vi "RH_DCPower_Configure.vi"(6 "output terminal":tag, 7 "DCPower_Parameters":T1={"Output"=enum."DC Voltage", "Current_range"=0.0, "Current"=0.0, "Voltage_range"=0.0, "Voltage"=0.0, "Aperture_time"=0.0, "Source Delay"=0.0, "Sense"=1008} {"Source Delay" format="%.6p"; "Sense" items=["Local"=1008, "Remote"=1009]; "Aperture_time" format="%.6p"; "Current_range" format="%.6p"; "Current" format="%.6p"; "Voltage_range" format="%.6p"; "Voltage" format="%.6p"}, 8 "error in (no error)":errorcluster, 9 "trigger out?":bool, 10 "channel name":string, 11 "DCPower Session In":refnum<k15>) -> (0 "error out":errorcluster, 3 "DCPower Session Out":refnum<k15>)   [LabVIEW 2023, in "ResourceHandling.lvlib"]
doc: "Config SMU/PS channel in DC Voltage or DC Current mode, exporting Start Trigger and setting the Aperture Time"
uses:
  ResourceHandling.lvlib
  TypeDefs/RH_DCPower_Parameters.ctl
  <instrlib>/niDCPower/nidcpower.llb/niDCPower Source Mode.ctl
  <instrlib>/niDCPower/nidcpower.llb/niDCPower Output Function.ctl
  <instrlib>/niDCPower/nidcpower.llb/niDCPower Export Signal - Signal.ctl
  <instrlib>/niDCPower/nidcpower.llb/niDCPower Aperture Time Units.ctl
  <instrlib>/niDCPower/nidcpower.llb/niDCPower Disable Start Trigger With Channels.vi
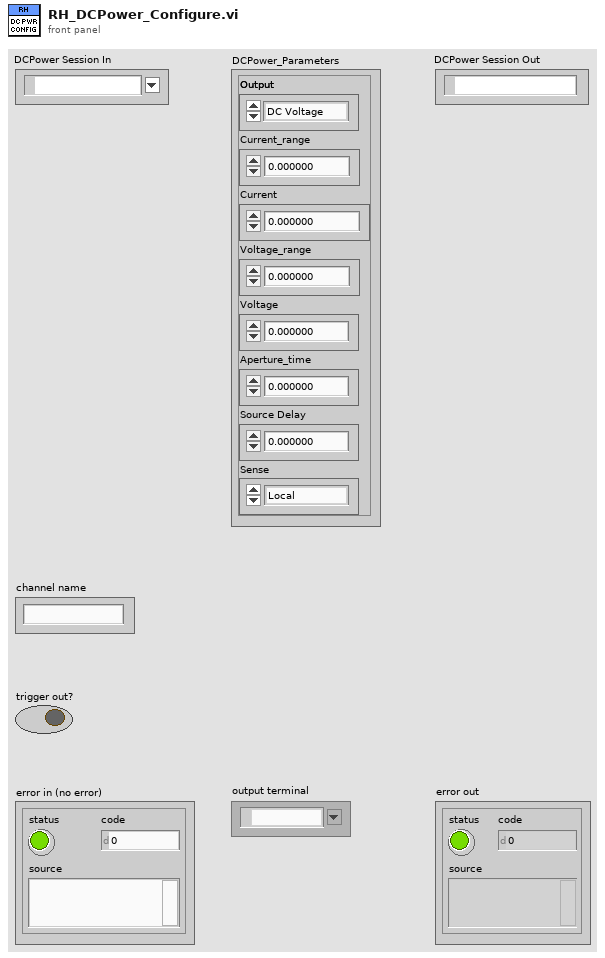
[diagram p1: front panel]
types:
  T1 = typedef "ResourceHandling.lvlib/RH_DCPower_Parameters.ctl" = cluster{"Output":enum16{"DC Voltage", "DC Current"}, "Current_range":dbl, "Current":dbl, "Voltage_range":dbl, "Voltage":dbl, "Aperture_time":dbl, "Source Delay":dbl, "Sense":i32}
  T2 = typedef "niDCPower Source Mode.ctl" = i32
  T3 = typedef "niDCPower Output Function.ctl" = i32
  T4 = typedef "niDCPower Export Signal - Signal.ctl" = i32
  T5 = typedef "niDCPower Aperture Time Units.ctl" = i32
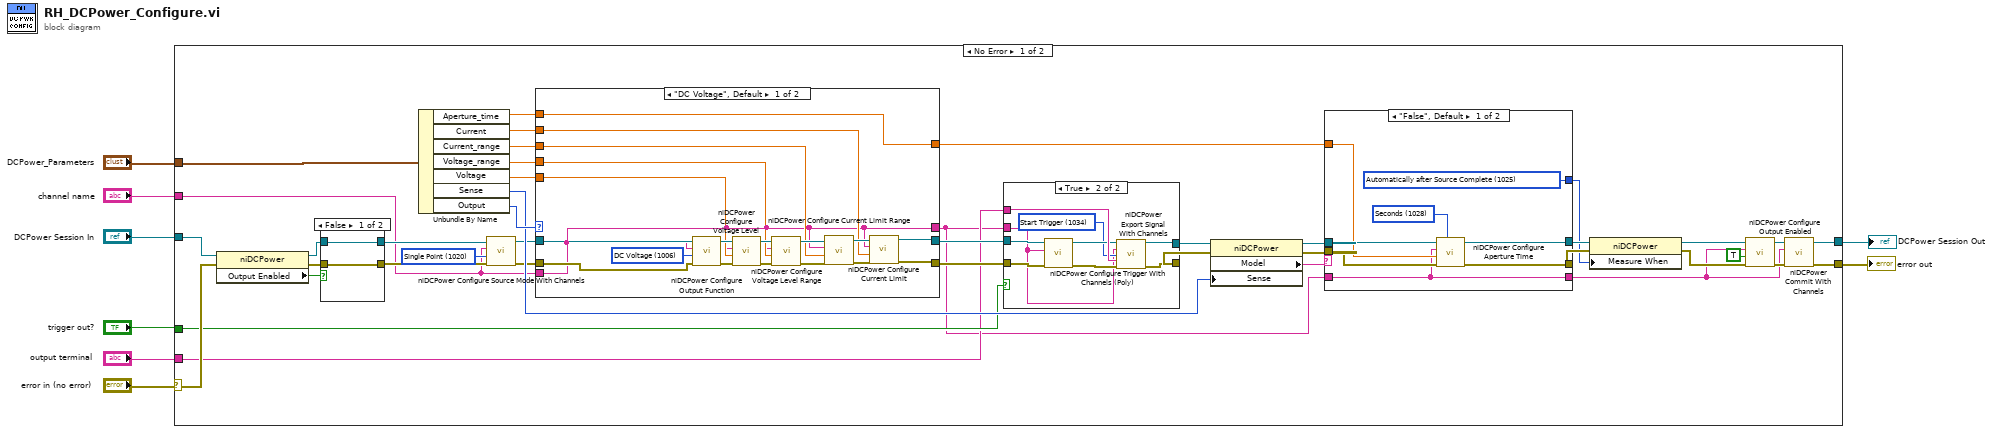
[diagram p0: block diagram]
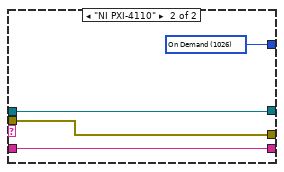
[diagram p2: hidden frame]
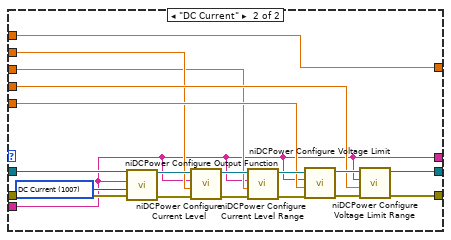
[diagram p4: hidden frame]
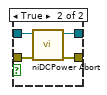
[diagram p5: hidden frame]
diagram:
  n1 = case shown="No Error" "error in (no error)" {
    selector: "error in (no error)" -> [w31 w118]
    tunnel: "DCPower_Parameters" -> [w35 _]
    tunnel: "DCPower Session In" -> [w34 w117]
    tunnel: [w33 w117] -> w1
    tunnel: [w32 w118] -> w7
    tunnel: "channel name" -> [w10 _]
    tunnel: "trigger out?" -> [w19 _]
    tunnel: "output terminal" -> [w18 _]
    frame No Error {
      w24 = T2 1020 items=["Single Point"=1020, "Sequence"=1021] ("source mode")
      n2 = property class="niDCPower"(reference=w34, error in=w31) -> (reference out=w48:refnum<k15>, error out=w49:errorcluster, "Output Enabled"=w47:bool)
      n3 = case shown="False" w47 {
        tunnel: w48 -> [w112 w116]
        tunnel: w49 -> [w111 w115]
        tunnel: [w112 w114] -> w28
        tunnel: [w111 w113] -> w26
        frame False {
        }
        frame True {
          n4 = call <instrlib>:"niDCPower Abort.vi"("error in (no error)"=w115, "instrument handle"=w116) -> ("error out"=w113:errorcluster, "instrument handle out"=w114:refnum<k15>)  [unwired: 8 in]
        }
      }
      n5 = Unbundle By Name(w35) -> ("Aperture_time"=w40:dbl, "Current"=w41:dbl, "Current_range"=w42:dbl, "Voltage_range"=w43:dbl, "Voltage"=w44:dbl, "Sense"=w29:i32, "Output"=w30:enum16{"DC Voltage", "DC Current"})
      n6 = call <instrlib>:"niDCPower Configure Source Mode With Channels.vi"("error in (no error)"=w26, "source mode"=w24, "channel name"=w10, "instrument handle"=w28) -> ("error out"=w25:errorcluster, "instrument handle out"=w27:refnum<k15>)  [unwired: 6 in]
      n7 = case shown="\"DC Voltage\", Default" w30 {
        tunnel: w25 -> [w82 w102]
        tunnel: w27 -> [w83 w101]
        tunnel: [w76 w97] -> w23
        tunnel: [w75 w96] -> w21
        tunnel: w44 -> [w86 w98]
        tunnel: w43 -> [w85 w99]
        tunnel: w42 -> [w79 w93]
        tunnel: w41 -> [w74 w94]
        tunnel: w40 -> [w84 w95]
        tunnel: [w84 w95] -> w36
        tunnel: w10 -> [w73 w92]
        tunnel: [w73 w92] -> w12
        frame "DC Voltage", Default {
          w87 = T3 1006 items=["DC Voltage"=1006, "DC Current"=1007, "Pulse Voltage"=1049, "Pulse Current"=1050] ("output function")
          n8 = call <instrlib>:"niDCPower Configure Output Function.vi"("error in (no error)"=w82, "output function"=w87, "channel name"=w73, "instrument handle"=w83) -> ("error out"=w89:errorcluster, "instrument handle out"=w88:refnum<k15>)  [unwired: 6 in]
          n9 = call <instrlib>:"niDCPower Configure Voltage Level.vi"("error in (no error)"=w89, "voltage level"=w86, "channel name"=w73, "instrument handle"=w88) -> ("error out"=w91:errorcluster, "instrument handle out"=w90:refnum<k15>)  [unwired: 6 in]
          n10 = call <instrlib>:"niDCPower Configure Voltage Level Range.vi"("error in (no error)"=w91, "voltage level range"=w85, "channel name"=w73, "instrument handle"=w90) -> ("error out"=w81:errorcluster, "instrument handle out"=w80:refnum<k15>)  [unwired: 6 in]
          n11 = call <instrlib>:"niDCPower Configure Current Limit Range.vi"("error in (no error)"=w81, "current limit range"=w79, "channel name"=w73, "instrument handle"=w80) -> ("error out"=w78:errorcluster, "instrument handle out"=w77:refnum<k15>)  [unwired: 6 in]
          n12 = call <instrlib>:"niDCPower Configure Current Limit.vi"("error in (no error)"=w78, "current limit"=w74, "channel name"=w73, "instrument handle"=w77) -> ("error out"=w75:errorcluster, "instrument handle out"=w76:refnum<k15>)  [unwired: 6 in]
        }
        frame "DC Current" {
          w100 = T3 1007 items=["DC Voltage"=1006, "DC Current"=1007, "Pulse Voltage"=1049, "Pulse Current"=1050] ("output function")
          n13 = call <instrlib>:"niDCPower Configure Output Function.vi"("error in (no error)"=w102, "output function"=w100, "channel name"=w92, "instrument handle"=w101) -> ("error out"=w103:errorcluster, "instrument handle out"=w104:refnum<k15>)  [unwired: 6 in]
          n14 = call <instrlib>:"niDCPower Configure Current Level.vi"("error in (no error)"=w103, "current level"=w94, "channel name"=w92, "instrument handle"=w104) -> ("error out"=w110:errorcluster, "instrument handle out"=w109:refnum<k15>)  [unwired: 6 in]
          n15 = call <instrlib>:"niDCPower Configure Current Level Range.vi"("error in (no error)"=w110, "current level range"=w93, "channel name"=w92, "instrument handle"=w109) -> ("error out"=w108:errorcluster, "instrument handle out"=w107:refnum<k15>)  [unwired: 6 in]
          n16 = call <instrlib>:"niDCPower Configure Voltage Limit.vi"("error in (no error)"=w108, "voltage limit"=w98, "channel name"=w92, "instrument handle"=w107) -> ("error out"=w106:errorcluster, "instrument handle out"=w105:refnum<k15>)  [unwired: 6 in]
          n17 = call <instrlib>:"niDCPower Configure Voltage Limit Range.vi"("error in (no error)"=w106, "voltage limit range"=w99, "channel name"=w92, "instrument handle"=w105) -> ("error out"=w96:errorcluster, "instrument handle out"=w97:refnum<k15>)  [unwired: 6 in]
        }
      }
      n18 = case shown="True" w19 {
        tunnel: w23 -> [w63 w69]
        tunnel: [w63 w72] -> w22
        tunnel: w21 -> [w62 w67]
        tunnel: [w62 w71] -> w20
        tunnel: w18 -> [_ w70]
        tunnel: w12 -> [_ w64]
        frame False {
        }
        frame True {
          w65 = T4 1034 items=["Source Complete Event"=1030, "Measure Complete Event"=1031, "Sequence Iteration Complete Event"=1032, "Sequence Engine Done Event"=1033, "Pulse Complete Event"=1051, "Ready For Pulse Trigger Event"=1052, "Start Trigger"=1034, "Source Trigger"=1035, "Measure Trigger"=1036, "Sequence Advance Trigger"=1037, "Pulse Trigger"=1053] ("signal")
          n19 = call-poly <instrlib>:"niDCPower Configure Trigger With Channels (Poly).vi"("error in (no error)"=w67, "channel name"=w64, "instrument handle"=w69) -> ("error out"=w66:errorcluster, "instrument handle out"=w68:refnum<k15>)  [unwired: 7 in]
          n20 = call <instrlib>:"niDCPower Export Signal With Channels.vi"("instrument handle"=w68, "channel name"=w64, "signal"=w65, "output terminal"=w70, "error in (no error)"=w66) -> ("instrument handle out"=w72:refnum<k15>, "error out"=w71:errorcluster)  [unwired: 9 in]
        }
      }
      n21 = property class="niDCPower"(reference=w22, error in=w20, "Sense"=w29) -> (reference out=w38:refnum<k15>, error out=w37:errorcluster, "Model"=w39:string)
      n22 = case shown="\"False\", Default" w39 {
        tunnel: w38 -> [w57 w61]
        tunnel: w37 -> [w56 w60]
        tunnel: [w55 w60] -> w16
        tunnel: [w54 w61] -> w17
        tunnel: w36 -> [w53 _]
        tunnel: w12 -> [w51 w59]
        tunnel: [w51 w59] -> w11
        tunnel: [w50 w58] -> w13
        frame "False", Default {
          w50 = 1025 items=["Automatically after Source Complete"=1025, "On Demand"=1026, "On Measure Trigger"=1027] ("Measurement:Advanced:Measure When")
          w52 = T5 1028 items=["Seconds"=1028, "Powerline Cycles"=1029] ("aperture time units")
          n23 = call <instrlib>:"niDCPower Configure Aperture Time.vi"("aperture time units"=w52, "error in (no error)"=w56, "aperture time"=w53, "channel name"=w51, "instrument handle"=w57) -> ("error out"=w55:errorcluster, "instrument handle out"=w54:refnum<k15>)  [unwired: 5 in]
        }
        frame "NI PXI-4110" {
          w58 = 1026 items=["Automatically after Source Complete"=1025, "On Demand"=1026, "On Measure Trigger"=1027] ("Measurement:Advanced:Measure When")
        }
      }
      n24 = property class="niDCPower"(reference=w17, error in=w16, "Measure When"=w13) -> (reference out=w14:refnum<k15>, error out=w15:errorcluster)
      n25 = call <instrlib>:"niDCPower Configure Output Enabled.vi"("error in (no error)"=w15, "output enabled"=TRUE, "channel name"=w11, "instrument handle"=w14) -> ("error out"=w46:errorcluster, "instrument handle out"=w45:refnum<k15>)  [unwired: 6 in]
      n26 = call <instrlib>:"niDCPower Commit With Channels.vi"("error in (no error)"=w46, "channel name"=w11, "instrument handle"=w45) -> ("error out"=w32:errorcluster, "instrument handle out"=w33:refnum<k15>)  [unwired: 7 in]
    }
    frame Error {
    }
  }
  "error out" <- w7
  "DCPower Session Out" <- w1
